vi "실습 3-2 난수일치.vi"() -> ()   [LabVIEW 2014]
panel:
  out "x+1":i32
  in  "숫자형":dbl min=0.0 max=10000.0 step=1.0
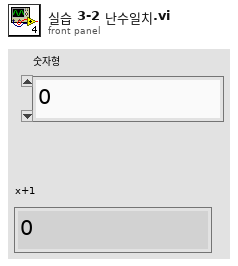
[diagram p1: front panel]
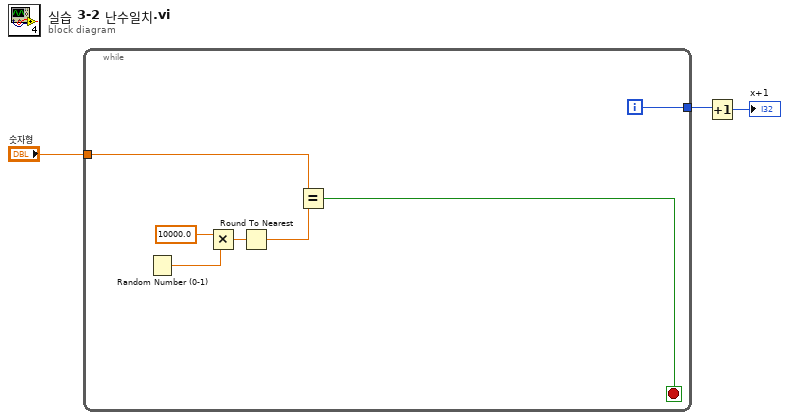
[diagram p0: block diagram]
diagram:
  n1 = while {
    tunnel: [w5] -> w3
    tunnel: "숫자형" -> [w4]
    i -> [w5]
    stop <- w9 stop-if-true
    n2 = Random Number (0-1)() -> (number: 0 to 1=w10:dbl)
    n3 = Multiply(x=10000.0, y=w10) -> (x*y=w8:dbl)
    n4 = Round To Nearest(number=w8) -> (nearest integer value=w6:dbl)
    n5 = Equal?(x=w4, y=w6) -> (x = y?=w9:bool)
  }
  n6 = Increment(x=w3) -> (x+1=→"x+1":i32)
